vi "ReceiveData.vi"(8 "error in (no error)":errorcluster, 10 "Input":string, 11 "Axis in":refnum<class "Axis.lvclass">) -> (0 "error out":errorcluster, 3 "Axis out":refnum<class "Axis.lvclass">)   [LabVIEW 2019, in "Axis.lvclass"]
uses:
  Axis.lvclass
  Axis.lvclass/Axis.ctl
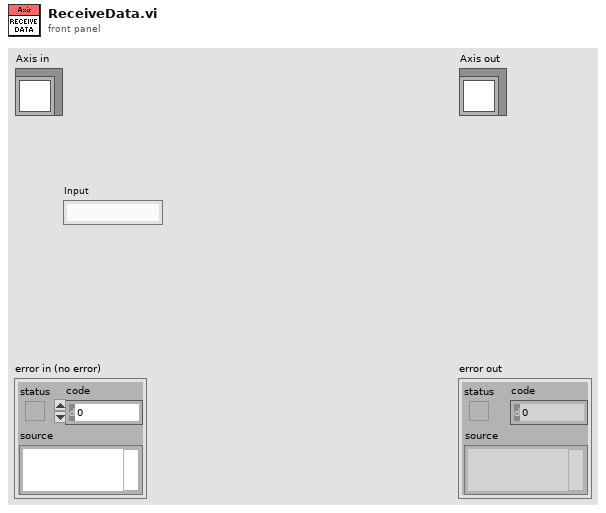
[diagram p1: front panel]
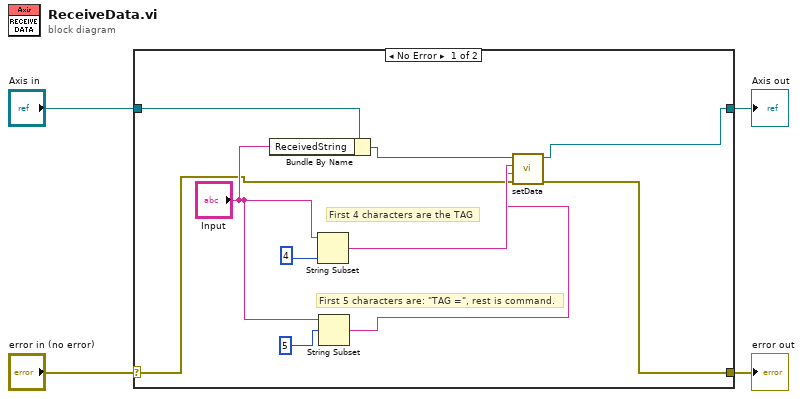
[diagram p0: block diagram]
diagram:
  n1 = case shown="No Error" "error in (no error)" {
    selector: "error in (no error)" -> [w6 w16]
    tunnel: [w5 w16] -> w3
    tunnel: [w9 w15] -> w1
    tunnel: "Axis in" -> [w14 w15]
    frame No Error {
      # "First 5 characters are: \"TAG =\", rest is command."
      # "First 4 characters are the TAG"
      n2 = Bundle By Name(cluster=w14, "ReceivedString"="Input") -> (w10:refnum<class "Axis.lvclass">)
      n3 = String Subset(string="Input", length (rest)=4) -> (substring=w8:string)  [unwired: 1 in]
      n4 = String Subset(string="Input", offset (0)=5) -> (substring=w7:string)  [unwired: 1 in]
      n5 = call-dynamic "setData.vi"("error in (no error)"=w6, "Value"=w7, "Tag"=w8, "Axis in"=w10) -> ("error out"=w5:errorcluster, "Axis out"=w9:refnum<class "Axis.lvclass">)  [unwired: 6 in]
    }
    frame Error {
    }
  }
  "error out" <- w3
  "Axis out" <- w1
